vi "4-7.vi"() -> (0 "猜测次数":i32, 1 "随机的数":i32)   [LabVIEW 2017]
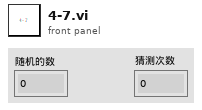
[diagram p1: front panel]
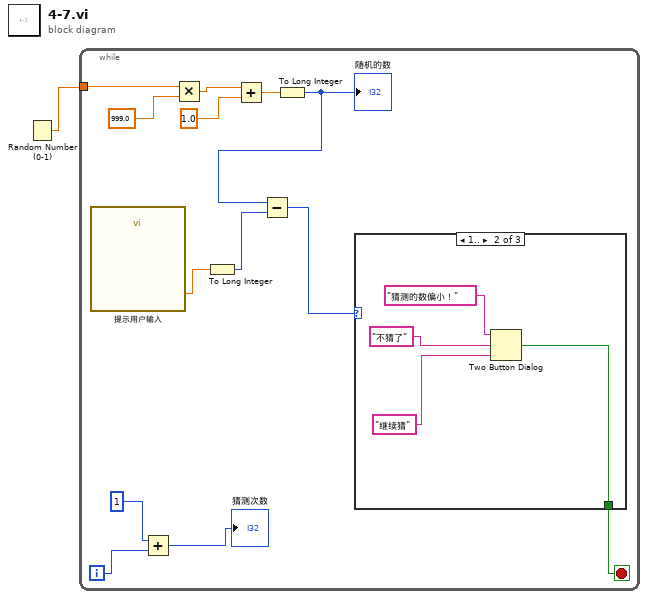
[diagram p0: block diagram]
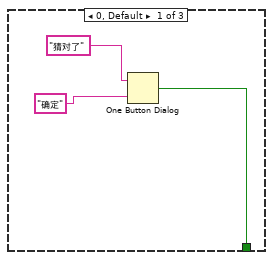
[diagram p2: hidden frame]
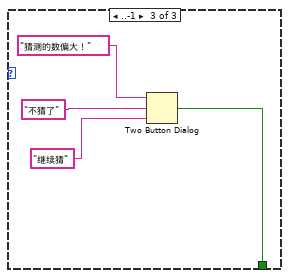
[diagram p3: hidden frame]
diagram:
  n1 = Random Number (0-1)() -> (number: 0 to 1=w1:dbl)
  n2 = while {
    tunnel: w1 -> [w2]
    i -> [w3]
    stop <- w6 stop-if-true
    n3 = call "提示用户输入"() -> ("请在1-1000猜"=w8:dbl)  [unwired: 17 in, 2 out]
    n4 = Add(x=1, y=w3) -> (x+y=→"猜测次数":i32)
    n5 = Multiply(x=w2, y=999.0) -> (x*y=w13:dbl)
    n6 = To Long Integer(number=w8) -> (32bit integer=w7:i32)
    n7 = Add(x=w13, y=1.0) -> (x+y=w11:dbl)
    n8 = To Long Integer(number=w11) -> (32bit integer=w10:i32)
    "随机的数" <- w10
    n9 = Subtract(x=w10, y=w7) -> (x-y=w9:i32)
    n10 = case shown="1.." w9 {
      tunnel: [w15 w18 w22] -> w6
      frame 0, Default {
        n11 = One Button Dialog(message="猜对了", button name ("OK")="确定") -> (true=w15:bool)
      }
      frame 1.. {
        n12 = Two Button Dialog(message="猜测的数偏小！", 1:"继续猜", 2:"不猜了") -> (T button?=w18:bool)
      }
      frame ..-1 {
        n13 = Two Button Dialog(message="猜测的数偏大！", 1:"继续猜", 2:"不猜了") -> (T button?=w22:bool)
      }
    }
  }
